vi "Read Data (Dictionary).vi"(8 "error in (no error)":errorcluster, 11 "LVtoITX in":refnum<class "LV to ITX.lvclass">) -> (0 "error out":errorcluster, 3 "LVtoITX out":refnum<class "LV to ITX.lvclass">)   [LabVIEW 2016, in "LV to ITX.lvclass"]
uses:
  LV to ITX.lvclass
  LV to ITX.lvclass/LV to ITX.ctl
panel:
  out "Data (Dictionary)":cluster{"key":variant, "value":variant}[](array[cluster])
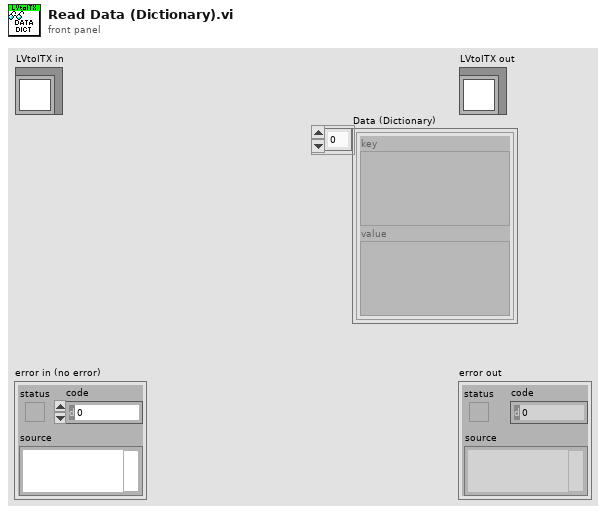
[diagram p1: front panel]
types:
  T1 = typedef "LV to ITX.lvclass/Dictionary--cluster.ctl" = cluster{"key":string, "value":variant}
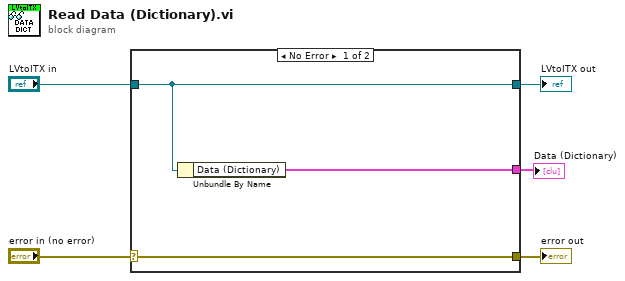
[diagram p0: block diagram]
diagram:
  n1 = case shown="No Error" "error in (no error)" {
    selector: "error in (no error)" -> [w8 w9]
    tunnel: [w8 w9] -> w4
    tunnel: [w7 w10] -> w2
    tunnel: "LVtoITX in" -> [w7 w10]
    tunnel: [w6 _] -> w1
    frame No Error {
      n2 = Unbundle By Name(w7) -> ("Data (Dictionary)"=w6:T1[])
    }
    frame Error {
    }
  }
  "error out" <- w4
  "LVtoITX out" <- w2
  "Data (Dictionary)" <- w1
